vi "Meas Result Update Thermometer Status.vi"(6 "str ref":refnum<vi>, 8 "error in":errorcluster, 11 "thermo in":T1={"type"=enum."COMET Tx5xx (ethernet)", "comment"="", "tag"="", "refresh"=5.0, "IP"="", "port"=502, "VISA"="", "last readout"=timestamp(0 s since 1904-01-01), "TCP ref"=refnum, "VISA sess"="", "idn"="", "press"=0.0, "RH"=0.0, "temp"=0.0, "pres cor"=[], "RH cor"=[], "temp cor"=[], "try left"=0, "failed"=FALSE, "RTD set"=[], "RTD inv"=[], "range"=0.0, "net mode"=enum."MODBUS", "try fail"=enum."Stop trying - return NaN", "timeout [s]"=0.0, "max retries"=0, "sim t [deg]"=0.0, "status"=0} {"status" items=["ok", "retry", "failed"]; "RTD inv" format="%.1f"; "RTD set" format="%.1f"; "temp cor" format="%.1f"; "RH cor" format="%.1f"; "pres cor" format="%.1f"; "refresh" min=0.1 max=1000.0 format="%.2f"}) -> (0 "error out":errorcluster, 3 "thermo out":T1={"type"=enum."COMET Tx5xx (ethernet)", "comment"="", "tag"="", "refresh"=5.0, "IP"="", "port"=502, "VISA"="", "last readout"=timestamp(0 s since 1904-01-01), "TCP ref"=refnum, "VISA sess"="", "idn"="", "press"=0.0, "RH"=0.0, "temp"=0.0, "pres cor"=[], "RH cor"=[], "temp cor"=[], "try left"=0, "failed"=FALSE, "RTD set"=[], "RTD inv"=[], "range"=0.0, "net mode"=enum."MODBUS", "try fail"=enum."Stop trying - return NaN", "timeout [s]"=0.0, "max retries"=0, "sim t [deg]"=0.0, "status"=0} {"status" items=["ok", "retry", "failed"]; "RTD inv" format="%.1f"; "RTD set" format="%.1f"; "temp cor" format="%.1f"; "RH cor" format="%.1f"; "pres cor" format="%.1f"; "refresh" min=0.1 max=1000.0 format="%.2f"})   [LabVIEW 2020]
doc: "Updates status line with current reading data for thermometer."
uses:
  thermo/thermo.ctl
  thermo/thermo_types.ctl
  thermo/Thermometer Fail Action.ctl
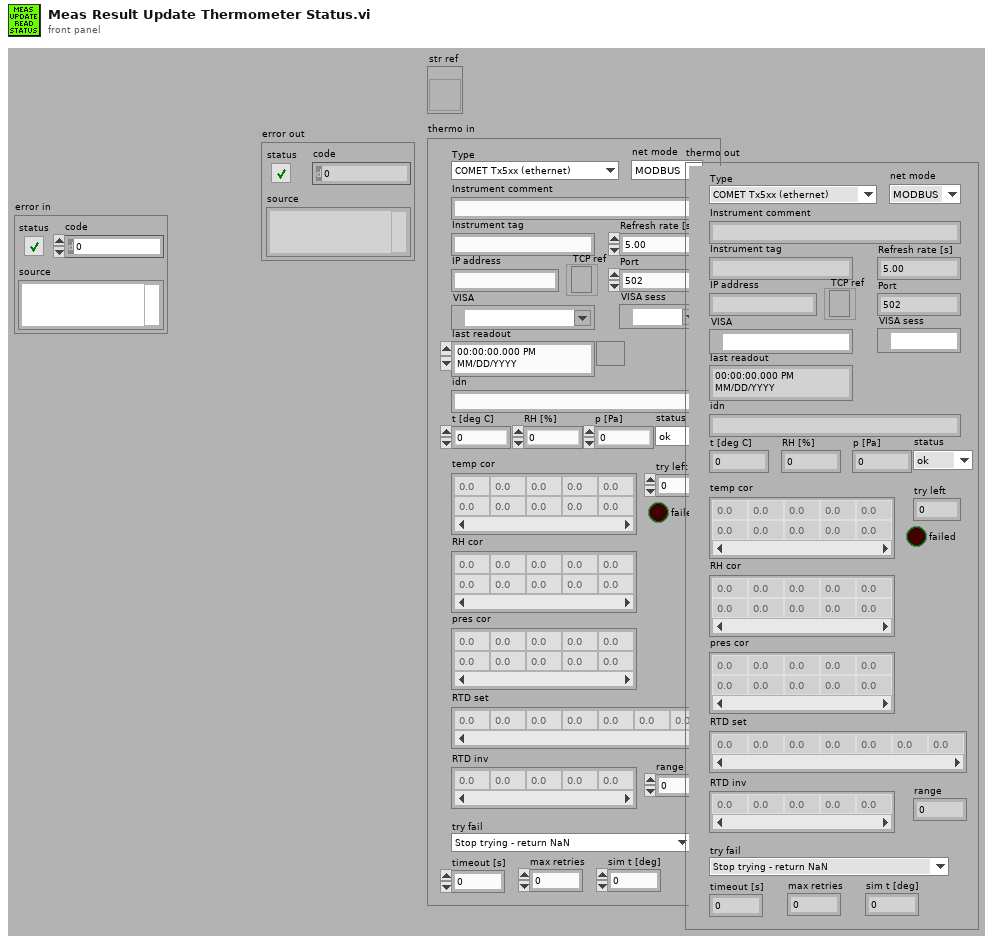
[diagram p1: front panel]
types:
  T1 = typedef "thermo.ctl" = cluster{"type":T2, "comment":string, "tag":string, "refresh":dbl, "IP":string, "port":u16, "VISA":refnum<visa-resource-name>, "last readout":timestamp, "TCP ref":refnum<k5>, "VISA sess":refnum<visa-resource-name>, "idn":string, "press":dbl, "RH":dbl, "temp":dbl, "pres cor":dbl[][], "RH cor":dbl[][], "temp cor":dbl[][], "try left":i32, "failed":bool, "RTD set":dbl[], "RTD inv":dbl[], "range":dbl, "net mode":enum16{"MODBUS", "HTTP"}, "try fail":T3, "timeout [s]":dbl, "max retries":i32, "sim t [deg]":dbl, "status":u16}
  T2 = typedef "thermo_types.ctl" = enum16{"Disabled", "Simulated", "COMET Tx5xx (ethernet)", "Keithley 2002 (GPIB) + RTD", "Agilent 344xx (GPIB) + RTD"}
  T3 = typedef "Thermometer Fail Action.ctl" = enum16{"Stop trying - keep last value", "Stop trying - return NaN", "Generate error - stop sweep"}
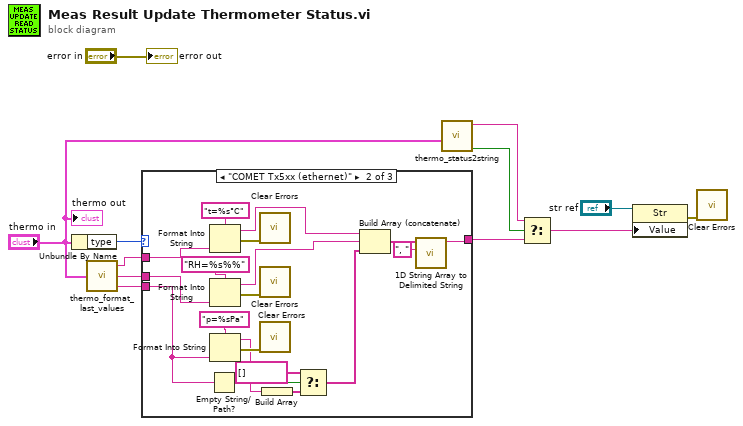
[diagram p0: block diagram]
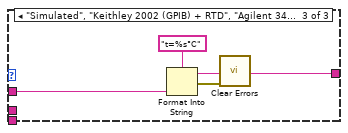
[diagram p3: hidden frame]
diagram:
  n1 = Unbundle By Name("thermo in") -> ("type"=w9:T2)
  n2 = call "thermo_format_last_values.vi"("thermo"="thermo in") -> ("temperature"=w8:string, "RH"=w7:string, "pressure"=w6:string)  [unwired: 4 in]
  n3 = case shown="\"COMET Tx5xx (ethernet)\"" w9 {
    tunnel: [_ w19 w33] -> w2
    tunnel: w8 -> [_ w30 w34]
    tunnel: w7 -> [_ w26 _]
    tunnel: w6 -> [_ w16 _]
    frame Default {
    }
    frame "COMET Tx5xx (ethernet)" {
      n4 = Empty String/Path?(string/path=w16) -> (empty?=w18:bool)
      n5 = Format Into String(format string="t=%s°C", w30) -> (resulting string=w23:string, error out=w29:errorcluster)  [unwired: 2 in]
      n6 = Format Into String(format string="RH=%s%%", w26) -> (resulting string=w22:string, error out=w28:errorcluster)  [unwired: 2 in]
      n7 = Format Into String(format string="p=%sPa", w16) -> (resulting string=w17:string, error out=w24:errorcluster)  [unwired: 2 in]
      n8 = call <vilib>:"Clear Errors.vi"("error in (no error)"=w29) -> ()  [unwired: 5 in, 2 out]
      n9 = call <vilib>:"Clear Errors.vi"("error in (no error)"=w28) -> ()  [unwired: 5 in, 2 out]
      n10 = call <vilib>:"Clear Errors.vi"("error in (no error)"=w24) -> ()  [unwired: 5 in, 2 out]
      n11 = Build Array(w17) -> (w14:string[])
      n12 = Select(t=string[] [], s=w18, f=w14) -> (s? t:f=w15:string[])
      n13 = Build Array (concatenate)(w23, w22, w15) -> (w21:string[])
      n14 = call <vilib>:"1D String Array to Delimited String.vi"("delimiter"=", ", "string array"=w21) -> ("delimited string"=w19:string)  [unwired: 9 in]
    }
    frame "Simulated", "Keithley 2002 (GPIB) + RTD", "Agilent 344xx (GPIB) + RTD" {
      n15 = Format Into String(format string="t=%s°C", w34) -> (resulting string=w33:string, error out=w32:errorcluster)  [unwired: 2 in]
      n16 = call <vilib>:"Clear Errors.vi"("error in (no error)"=w32) -> ()  [unwired: 5 in, 2 out]
    }
  }
  n17 = call "thermo_status2string.vi"("thermo"="thermo in") -> ("message available"=w4:bool, "status string"=w3:string)  [unwired: 9 in]
  n18 = Select(t=w3, s=w4, f=w2) -> (s? t:f=w1:string)
  n19 = property class="Str"(reference="str ref", "Value"=w1) -> (error out=w10:errorcluster)  [unwired: 1 in, 1 out]
  n20 = call <vilib>:"Clear Errors.vi"("error in (no error)"=w10) -> ()  [unwired: 5 in, 2 out]
  "error out" <- "error in"
  "thermo out" <- "thermo in"
